vi "Generate version information from files and folders.vi"(8 "error in (no error)":errorcluster, 11 "selected path":path) -> (0 "error out":errorcluster, 1 "Array":string[][](array[string]), 2 "Numeric Control":i32, 3 "file paths":path[](array[path]))   [LabVIEW 2014]
panel:
  out "Numeric Control 2":i32
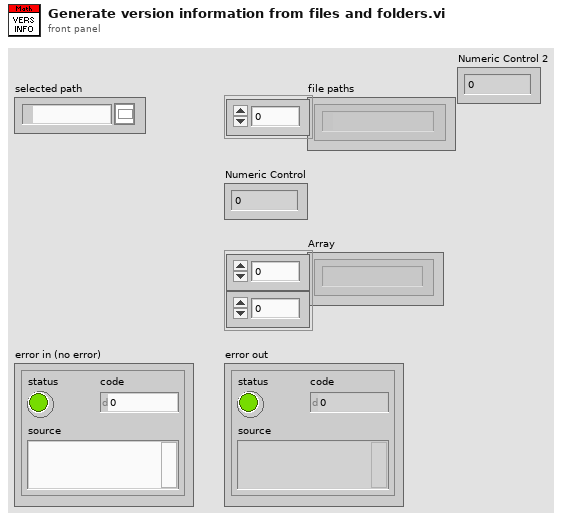
[diagram p1: front panel]
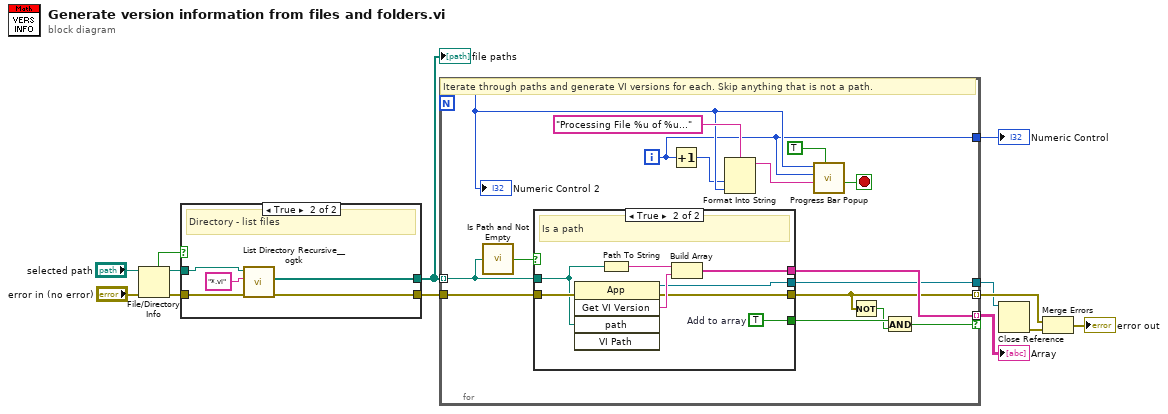
[diagram p0: block diagram]
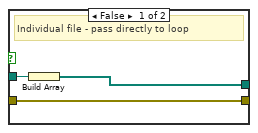
[diagram p2: hidden frame]
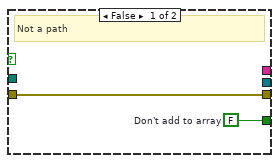
[diagram p3: hidden frame]
diagram:
  n1 = File/Directory Info(path="selected path", error in="error in (no error)") -> (path out=w11:path, directory=w6:bool, error out=w7:errorcluster)  [unwired: 4 out]
  n2 = case shown="True" w6 {
    tunnel: [w15 w20] -> w13
    tunnel: w11 -> [w16 w21]
    tunnel: w7 -> [w14 w19]
    tunnel: [w14 w18] -> w8
    frame False {
      # "Individual file - pass directly to loop"
      n3 = Build Array(w16) -> (w15:path[])
    }
    frame True {
      # "Directory - list files"
      n4 = call <userlib>:"List Directory Recursive__ogtk.vi"("error in (no error)"=w19, "pattern"="*.vi", "Path"=w21) -> ("error out"=w18:errorcluster, "file paths"=w20:path[])  [unwired: 5 in, 2 out]
    }
  }
  "file paths" <- w13
  n5 = for {
    N -> [w24]
    tunnel: [w37] -> w5 mode=indexing if=w29
    tunnel: [w36] -> w1
    tunnel: [w31] -> w2 mode=indexing
    tunnel: w13 -> [w34] mode=indexing
    tunnel: w8 -> [w33]
    tunnel: [w23] -> w12
    i -> [w23]
    stop <- w25 stop-if-true
    # "Iterate through paths and generate VI versions for each. Skip anything that is not a path."
    n6 = call <vilib>:"Is Path and Not Empty.vi"("path"=w34) -> ("Is Path and Not Empty?"=w35:bool)  [unwired: 4 in]
    n7 = case shown="True" w35 {
      tunnel: [_ w41] -> w37
      tunnel: [_ w46] -> w36
      tunnel: w34 -> [_ w42]
      tunnel: [w39 w45] -> w32
      tunnel: [w38 w44] -> w31
      tunnel: w33 -> [w38 w43]
      frame False {
        w39 = FALSE  # Don't add to array
        # "Not a path"
      }
      frame True {
        w45 = TRUE  # Add to array
        # "Is a path"
        n8 = invoke class="App" method="Get VI Version"(error in=w43, "path"=w42) -> (reference out=w46:refnum<vi>, error out=w44:errorcluster, "GetVIVers"=w47:string)  [unwired: 3 in, 2 out]
        n9 = Path To String(path=w42) -> (string=w40:string)
        n10 = Build Array(w40, w47) -> (w41:string[])
      }
    }
    n11 = Increment(x=w23) -> (x+1=w22:i32)
    n12 = Format Into String(format string="Processing File %u of %u..." ("Message (Please Wait...)"), w22, w24) -> (resulting string=w27:string)  [unwired: 2 in, 1 out]
    n13 = call "Progress Bar Popup.vi"("Abort visible? (T)"=TRUE, "Message (Please Wait...)"=w27, "Current Iteration"=w23, "Total Iterations"=w24) -> ("Aborted"=w25:bool)  [unwired: 7 in]
    n14 = Not(x=w31) -> (.not. x?=w30:bool)
    n15 = And(x=w32, y=w30) -> (x .and. y?=w29:bool)
    "Numeric Control 2" <- w24
  }
  "Numeric Control" <- w12
  "Array" <- w5
  n16 = Close Reference(reference=w1) -> (error out=w4:errorcluster)  [unwired: 1 in]
  n17 = Merge Errors(w2, w4) -> (→"error out":errorcluster)
